vi "HTTPMethod_Core.vi"(4 "cancellationToken":refnum<k24>, 5 "ReturnHeadersFirst":bool, 6 "HttpRequest":refnum<k24>, 7 "Method":T1, 8 "error in (no error)":errorcluster, 9 "HttpContent":refnum<k24>, 10 "uri":refnum<k24>, 11 "HttpClient":refnum<k24>) -> (0 "error out":errorcluster, 3 "HttpResponseMessage":refnum<k24>)   [LabVIEW 2018, in "HttpClient_NET.lvlib" / "HttpClient_NET.lvclass"]
uses:
  HttpClient_NET.lvclass
  System.Net.Http
  Types/method_enum.ctl
  Types/HttpNet_error_enum.ctl
  HttpClient_NET.lvlib
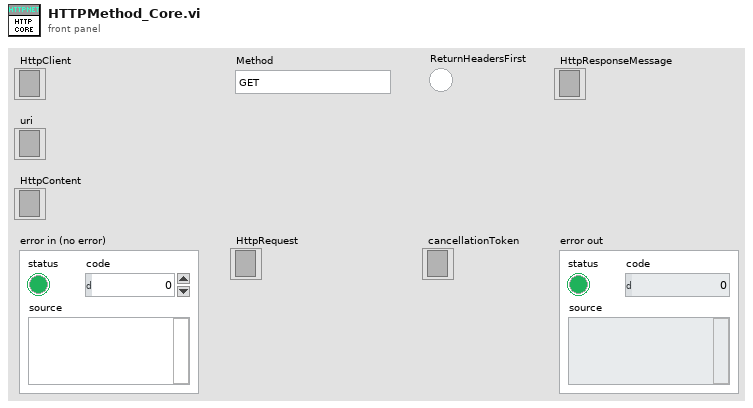
[diagram p1: front panel]
types:
  T1 = typedef "HttpClient_NET.lvlib/method_enum.ctl" = enum16{"GET", "PUT", "POST", "DELETE", "HEAD", "TRACE", "SEND"}
  T2 = typedef "HttpClient_NET.lvlib/HttpNet_error_enum.ctl" = enum16{"REST method is not available", "URL cannot be blank", "Output filepath cannot be empty", "Input filepath cannot be empty", "Internal .NET error %s", "Output filepath cannot be directory", "Download Task no longer exists", "Mutipart Put not supported from REST Client Interface.  Please revert to lower level classes"}
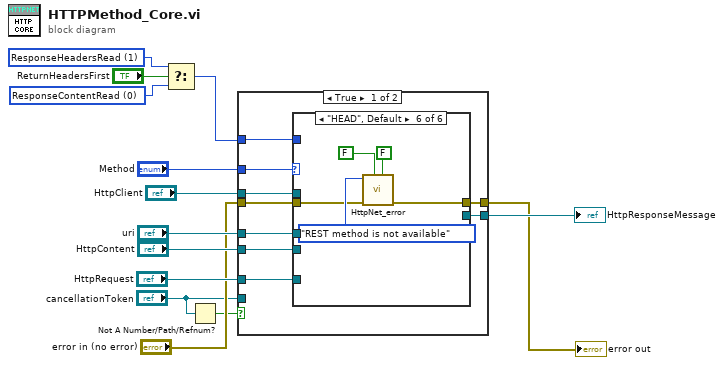
[diagram p0: block diagram]
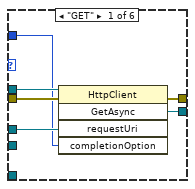
[diagram p2: hidden frame]
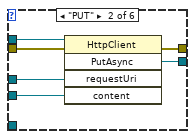
[diagram p3: hidden frame]
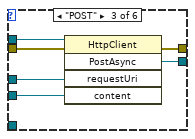
[diagram p4: hidden frame]
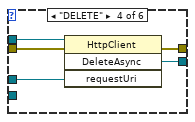
[diagram p5: hidden frame]
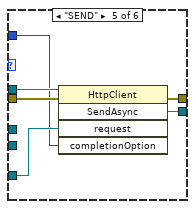
[diagram p6: hidden frame]
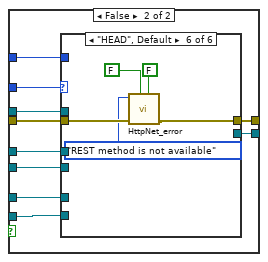
[diagram p7: hidden frame]
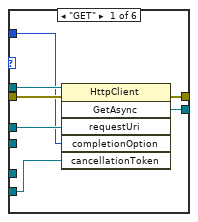
[diagram p8: hidden frame]
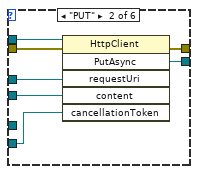
[diagram p9: hidden frame]
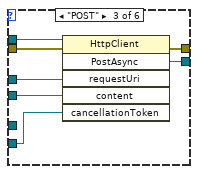
[diagram p10: hidden frame]
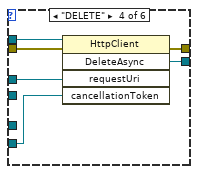
[diagram p11: hidden frame]
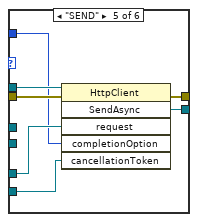
[diagram p12: hidden frame]
diagram:
  w3 = 1 items=["ResponseContentRead", "ResponseHeadersRead"] ("completionOption")
  w2 = 0 items=["ResponseContentRead", "ResponseHeadersRead"] ("completionOption")
  n1 = Select(t=w3, s="ReturnHeadersFirst", f=w2) -> (s? t:f=w1:i32)
  n2 = Not A Number/Path/Refnum?(number/path/refnum="cancellationToken") -> (NaN/Path/Refnum?=w6:bool)
  n3 = case shown="True" w6 {
    tunnel: [w23 w67] -> w14
    tunnel: [w22 w66] -> w13
    tunnel: "HttpRequest" -> [w21 w65]
    tunnel: "HttpContent" -> [w20 w64]
    tunnel: "uri" -> [w19 w63]
    tunnel: "error in (no error)" -> [w18 w62]
    tunnel: "Method" -> [w17 w61]
    tunnel: "HttpClient" -> [w16 w60]
    tunnel: "cancellationToken" -> [_ w59]
    tunnel: w1 -> [w15 w58]
    frame True {
      n4 = case shown="\"HEAD\", Default" w17 {
        tunnel: w16 -> [w29 w35 w41 w46 w52 _]
        tunnel: [w28 w30 w36 w42 w49 _] -> w23
        tunnel: w18 -> [w27 w34 w40 w45 w51 w53]
        tunnel: [w26 w33 w39 w44 w50 w55] -> w22
        tunnel: w19 -> [w25 w32 w38 w43 _ _]
        tunnel: w20 -> [_ w31 w37 _ _ _]
        tunnel: w21 -> [_ _ _ _ w48 _]
        tunnel: w15 -> [w24 _ _ _ w47 _]
        frame "GET" {
          n5 = invoke class="HttpClient" method="GetAsync"(reference=w29, error in=w27, "requestUri"=w25, "completionOption"=w24) -> (error out=w26:errorcluster, "GetAsync"=w28:refnum<k24>)  [unwired: 1 in, 3 out]
        }
        frame "PUT" {
          n6 = invoke class="HttpClient" method="PutAsync"(reference=w35, error in=w34, "requestUri"=w32, "content"=w31) -> (error out=w33:errorcluster, "PutAsync"=w30:refnum<k24>)  [unwired: 1 in, 3 out]
        }
        frame "POST" {
          n7 = invoke class="HttpClient" method="PostAsync"(reference=w41, error in=w40, "requestUri"=w38, "content"=w37) -> (error out=w39:errorcluster, "PostAsync"=w36:refnum<k24>)  [unwired: 1 in, 3 out]
        }
        frame "DELETE" {
          n8 = invoke class="HttpClient" method="DeleteAsync"(reference=w46, error in=w45, "requestUri"=w43) -> (error out=w44:errorcluster, "DeleteAsync"=w42:refnum<k24>)  [unwired: 1 in, 2 out]
        }
        frame "SEND" {
          n9 = invoke class="HttpClient" method="SendAsync"(reference=w52, error in=w51, "request"=w48, "completionOption"=w47) -> (error out=w50:errorcluster, "SendAsync"=w49:refnum<k24>)  [unwired: 1 in, 3 out]
        }
        frame "HEAD", Default {
          n10 = call "HttpNet_error.vi"("ShowCallChain [T]"=FALSE, "OverrideExistingErrors [T]"=FALSE, "Error In"=w53, "Error"=HttpNet_error_enum."REST method is not available") -> ("Error Out"=w55:errorcluster)  [unwired: 7 in]
        }
      }
    }
    frame False {
      n11 = case shown="\"HEAD\", Default" w61 {
        tunnel: w60 -> [w74 w81 w88 w94 w101 _]
        tunnel: [w73 w76 w83 w90 w98 _] -> w67
        tunnel: w62 -> [w72 w80 w87 w93 w100 w106]
        tunnel: [w71 w79 w86 w92 w99 w105] -> w66
        tunnel: w63 -> [w70 w78 w85 w91 _ _]
        tunnel: w64 -> [_ w77 w84 _ _ _]
        tunnel: w65 -> [_ _ _ _ w97 _]
        tunnel: w59 -> [w69 w75 w82 w89 w96 _]
        tunnel: w58 -> [w68 _ _ _ w95 _]
        frame "GET" {
          n12 = invoke class="HttpClient" method="GetAsync"(reference=w74, error in=w72, "requestUri"=w70, "completionOption"=w68, "cancellationToken"=w69) -> (error out=w71:errorcluster, "GetAsync"=w73:refnum<k24>)  [unwired: 1 in, 4 out]
        }
        frame "PUT" {
          n13 = invoke class="HttpClient" method="PutAsync"(reference=w81, error in=w80, "requestUri"=w78, "content"=w77, "cancellationToken"=w75) -> (error out=w79:errorcluster, "PutAsync"=w76:refnum<k24>)  [unwired: 1 in, 4 out]
        }
        frame "POST" {
          n14 = invoke class="HttpClient" method="PostAsync"(reference=w88, error in=w87, "requestUri"=w85, "content"=w84, "cancellationToken"=w82) -> (error out=w86:errorcluster, "PostAsync"=w83:refnum<k24>)  [unwired: 1 in, 4 out]
        }
        frame "DELETE" {
          n15 = invoke class="HttpClient" method="DeleteAsync"(reference=w94, error in=w93, "requestUri"=w91, "cancellationToken"=w89) -> (error out=w92:errorcluster, "DeleteAsync"=w90:refnum<k24>)  [unwired: 1 in, 3 out]
        }
        frame "SEND" {
          n16 = invoke class="HttpClient" method="SendAsync"(reference=w101, error in=w100, "request"=w97, "completionOption"=w95, "cancellationToken"=w96) -> (error out=w99:errorcluster, "SendAsync"=w98:refnum<k24>)  [unwired: 1 in, 4 out]
        }
        frame "HEAD", Default {
          n17 = call "HttpNet_error.vi"("ShowCallChain [T]"=FALSE, "OverrideExistingErrors [T]"=FALSE, "Error In"=w106, "Error"=HttpNet_error_enum."REST method is not available") -> ("Error Out"=w105:errorcluster)  [unwired: 7 in]
        }
      }
    }
  }
  "HttpResponseMessage" <- w14
  "error out" <- w13
